vi "Launch Set Up.vi"(8 "error in (no error)":errorcluster, 11 "name or relative path":string) -> (0 "error out":errorcluster, 3 "appended path":path)   [LabVIEW 2012]
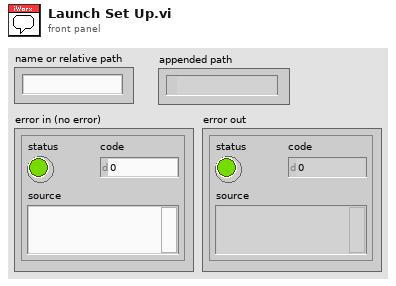
[diagram p1: front panel]
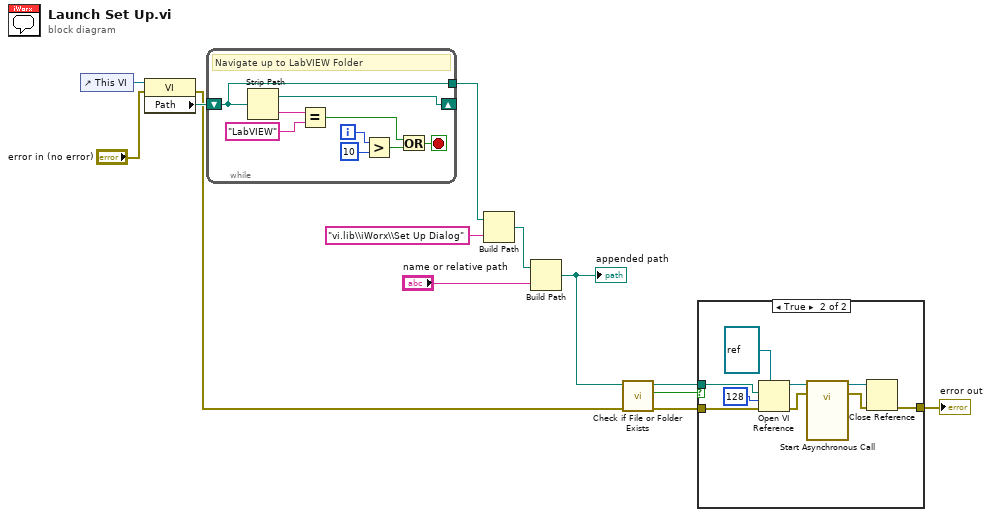
[diagram p0: block diagram]
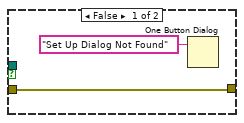
[diagram p2: hidden frame]
diagram:
  n1 = control-ref of="This VI"() -> (w8:refnum<vi>)
  n2 = property class="VI"(reference=w8, error in="error in (no error)") -> (error out=w5:errorcluster, "Path"=w9:path)  [unwired: 1 out]
  n3 = while {
    shift-right: [w22] -> _
    shift-left: w9 -> [w19]
    tunnel: [w19] -> w12
    i -> [w17]
    stop <- w14 stop-if-true
    # "Navigate up to LabVIEW Folder"
    n4 = Strip Path(path=w19) -> (stripped path=w22:path, name=w21:string)
    n5 = Equal?(x=w21, y="LabVIEW" ("name or relative path")) -> (x = y?=w18:bool)
    n6 = Greater?(x=w17, y=10) -> (0:w15:bool)
    n7 = Or(x=w18, y=w15) -> (x .or. y?=w14:bool)
  }
  n8 = Build Path(base path=w12, name or relative path="vi.lib\\iWorx\\Set Up Dialog") -> (appended path=w13:path)
  n9 = Build Path(base path=w13, name or relative path="name or relative path") -> (appended path=w4:path)
  "appended path" <- w4
  n10 = call <vilib>:"Check if File or Folder Exists.vi"("error in (no error)"=w5, "path"=w4) -> ("error out"=w2:errorcluster, "file or folder exists?"=w1:bool, "dup path"=w3:path)  [unwired: 7 in]
  n11 = case shown="True" w1 {
    tunnel: [w24 w32] -> w7
    tunnel: w3 -> [_ w26]
    tunnel: w2 -> [w24 w25]
    frame False {
      n12 = One Button Dialog(message="Set Up Dialog Not Found") -> ()  [unwired: 1 in, 1 out]
    }
    frame True {
      n13 = Open VI Reference(type specifier VI Refnum (for type only)=refnum<vi> refnum, vi path=w26, options=128, error in (no error)=w25) -> (vi reference=w31:refnum<vi>, error out=w28:errorcluster)  [unwired: 2 in]
      n14 = call-by-ref "Start Asynchronous Call"(reference=w31, error in=w28) -> (reference out=w30:refnum<vi>, error out=w29:errorcluster)  [unwired: 12 in]
      n15 = Close Reference(reference=w30, error in (no error)=w29) -> (error out=w32:errorcluster)
    }
  }
  "error out" <- w7
